vi "Remove Excess Rows.vi"(1 "Initial Array":dbl[][](array[numeric])) -> (0 "Truncated Array":dbl[][](array[numeric]))   [LabVIEW 2015]
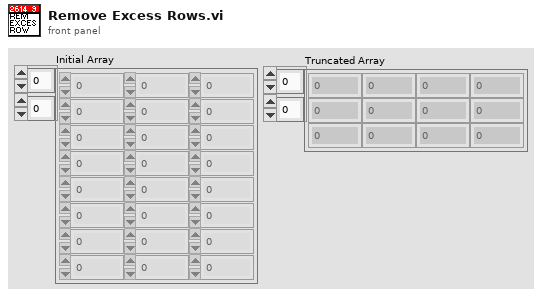
[diagram p1: front panel]
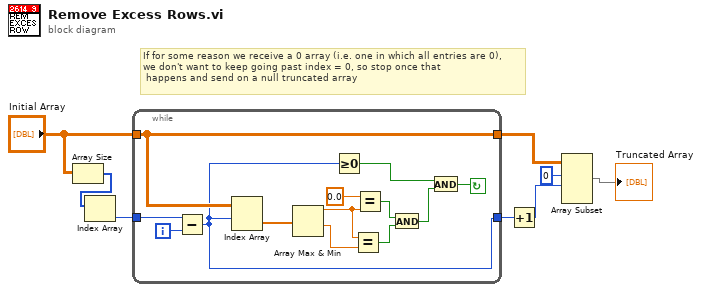
[diagram p0: block diagram]
diagram:
  # "If for some reason we receive a 0 array (i.e. one in which all entries are 0),\nwe don't want to keep going past index = 0, so stop once that\n happens and send on a null truncated array"
  n1 = Array Size(array="Initial Array") -> (size(s)=w7:i32[])
  n2 = Index Array(array=w7) -> (element=w6:i32)  [unwired: 1 in]
  n3 = while {
    tunnel: "Initial Array" -> [w13]
    tunnel: w6 -> [w21]
    tunnel: [w12] -> w2
    tunnel: [w13] -> w5
    i -> [w14]
    stop <- w9 continue-if-true
    n4 = Subtract(x=w21, y=w14) -> (x-y=w12:i32)
    n5 = Index Array(array=w13, index (row)=w12) -> (element=w20:dbl[])  [unwired: 1 in]
    n6 = Array Max & Min(array=w20) -> (max value=w18:dbl, min value=w17:dbl)  [unwired: 2 out]
    n7 = Greater Or Equal To 0?(x=w12) -> (x >= 0?=w11:bool)
    n8 = Equal?(x=w18, y=w17) -> (x = y?=w15:bool)
    n9 = Equal?(x=0.0, y=w18) -> (x = y?=w16:bool)
    n10 = And(x=w16, y=w15) -> (x .and. y?=w10:bool)
    n11 = And(x=w11, y=w10) -> (x .and. y?=w9:bool)
  }
  n12 = Increment(x=w2) -> (x+1=w1:i32)
  n13 = Array Subset(array=w5, index (row)=0 ("index"), length (row)=w1) -> (→"Truncated Array":dbl[][])  [unwired: 2 in]
